vi "Waveform Data Averager.vi"(7 "Samples Per Average":i32, 10 "V to AU Conversion":dbl, 11 "Voltage Array In":dbl[](array[numeric])) -> (2 "AU Array Out":dbl[](array[numeric]), 3 "Voltage Array Out":dbl[](array[numeric]))   [LabVIEW 2016]
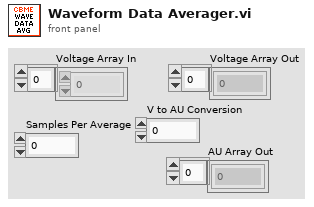
[diagram p1: front panel]
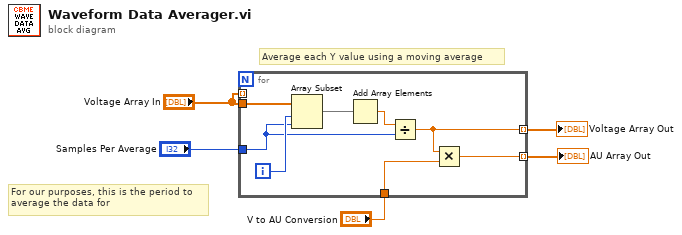
[diagram p0: block diagram]
diagram:
  # "Average each Y value using a moving average"
  # "For our purposes, this is the period to\naverage the data for"
  n1 = for {
    tunnel: "Voltage Array In" -> [_] mode=indexing
    tunnel: "Voltage Array In" -> [w13]
    tunnel: "Samples Per Average" -> [w9]
    tunnel: [w8] -> w5 mode=indexing
    tunnel: "V to AU Conversion" -> [w7]
    tunnel: [w6] -> w1 mode=indexing
    i -> [w12]
    n2 = Array Subset(array=w13, index=w12, length=w9) -> (w11:dbl[])
    n3 = Add Array Elements(numeric array=w11) -> (sum=w10:dbl)
    n4 = Divide(x=w10, y=w9) -> (x/y=w8:dbl)
    n5 = Multiply(x=w8, y=w7) -> (x*y=w6:dbl)
  }
  "Voltage Array Out" <- w5
  "AU Array Out" <- w1
